vi "ev3-samplecollector.vi"() -> ()   [LabVIEW 2013]
uses:
  <vilib>/Utility/inputDevices.llb/joystickAcquire.vi
  <vilib>/NXT/Dual Mode Library/Sensors/Read_Battery.vi
  <vilib>/NXT/Block Support/NXT_OutputPort.ctl
  <vilib>/NXT/LegoClasses/BrickReference/BrickReference.lvclass
  <vilib>/NXT/Subs/LVHSConnector.ctl
  <vilib>/NXT/NXTIO Xnodes/NXTIONodeSubVIs/NXTMoveMotors.vi
  <vilib>/NXT/NXTIO Xnodes/NXTIOXNode/NXTIO.xnode
  <vilib>/NXT/Dual Mode Library/Sound/Tone.vi
  <vilib>/Utility/inputDevices.llb/closeJoystick.vi
  <vilib>/NXT/NXTIO Xnodes/NXTIONodeSubVIs/NXTStopMotors.vi
  <vilib>/NXT/NXTIO Xnodes/AddressXNode/NXTIOAddress.xnode
  <vilib>/NXT/NXT Controls/ConnectionType.ctl
panel:
  in  "Connection Type":T1=enum."USB"
  in  "NXT/EV3 name":string
  out "throttle":dbl(knob) scale=0.0..100.0
  in  "Stop Button":bool
  out "Battery voltage [V]":sgl(slide) scale=0.0..10.0
  in  "Enable throttle":bool
  out "Voltage":dbl
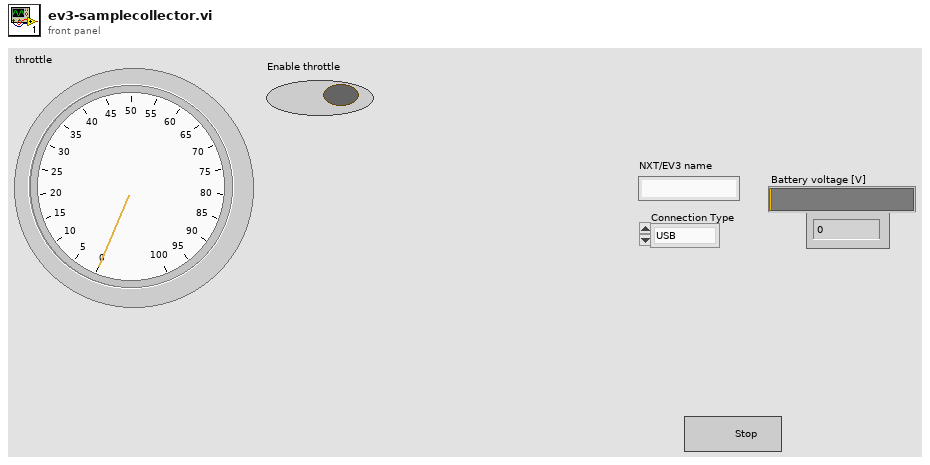
[diagram p1: front panel]
types:
  T1 = typedef "ConnectionType.ctl" = enum16{"Bluetooth", "USB", "WiFi"}
  T2 = typedef "LVHSConnector.ctl" = refnum<class "BrickReference.lvclass">
  T3 = typedef "NXT_OutputPort.ctl" = u8
  T4 = cluster{"X axis":i32, "Y axis":i32, "Z axis":i32, "X axis rotation":i32, "Y axis rotation":i32, "Z axis rotation":i32, "U axis":i32, "V axis":i32}
  T5 = cluster{"button 1":bool, "button 2":bool, "button 3":bool, "button 4":bool, "button 5":bool, "button 6":bool, "button 7":bool, "button 8":bool, "button 9":bool, "button 10":bool, "button 11":bool, "button 12":bool, "button 13":bool, "button 14":bool, "button 15":bool, "button 16":bool, "button 17":bool, "button 18":bool, "button 19":bool, "button 20":bool, "button 21":bool, "button 22":bool, "button 23":bool, "button 24":bool, "button 25":bool, "button 26":bool, "button 27":bool, "button 28":bool, "button 29":bool, "button 30":bool, "button 31":bool, "button 32":bool}
  T6 = cluster{"X axis":dbl, "Y axis":dbl, "Z axis":dbl, "X axis rotation":dbl, "Y axis rotation":dbl, "Z axis rotation":dbl, "U axis":dbl, "V axis":dbl}
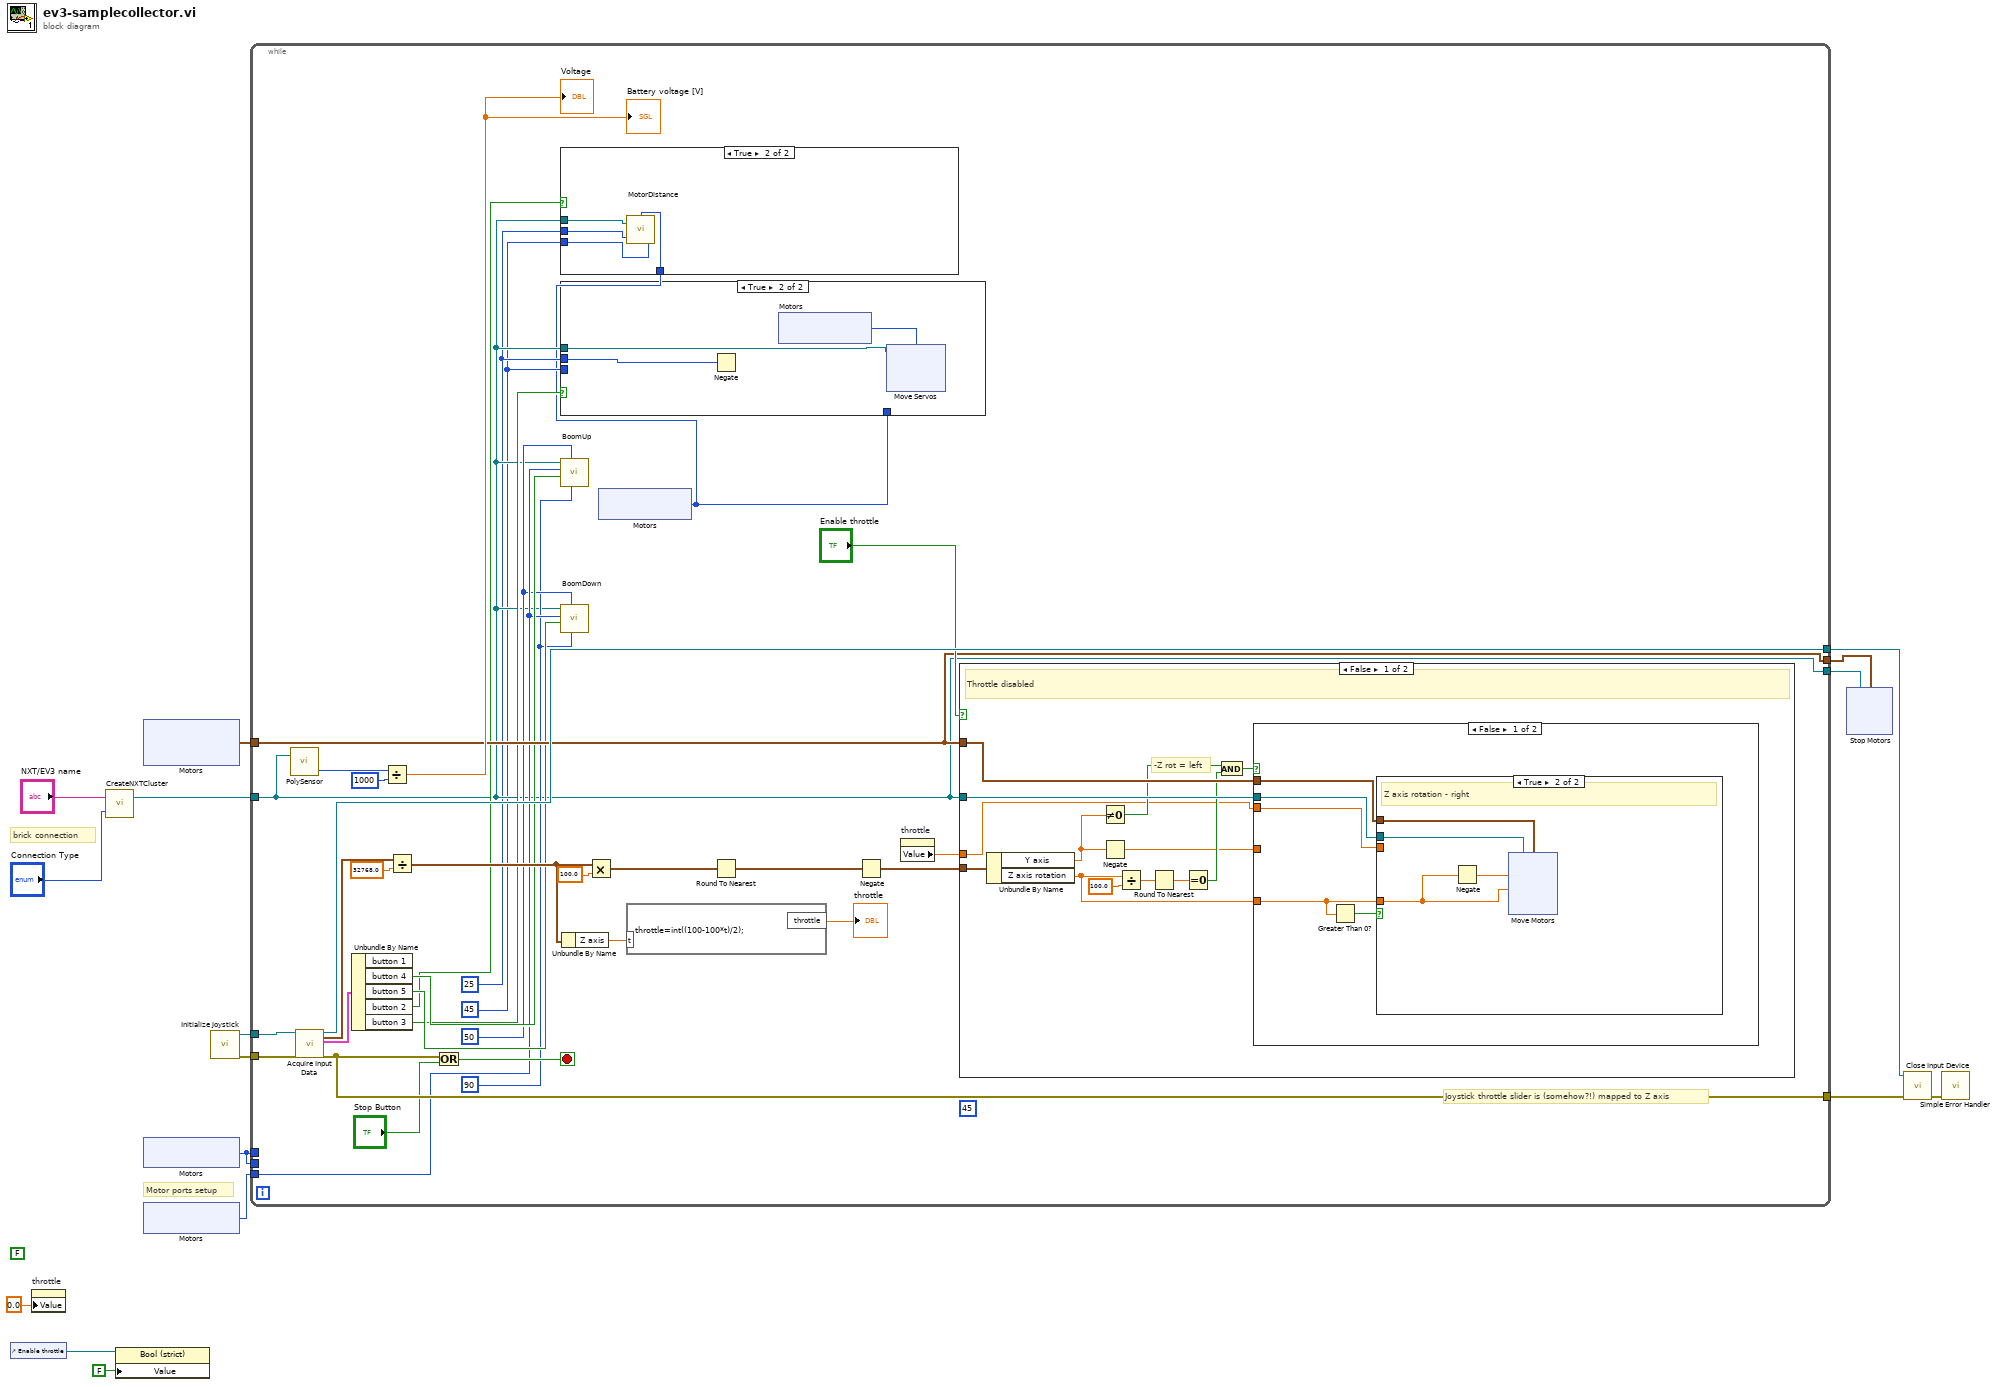
[diagram p0: block diagram]
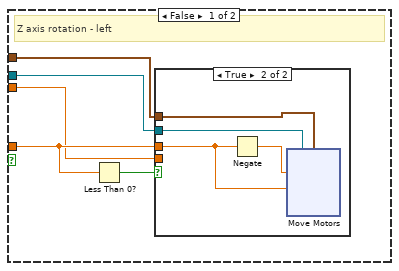
[diagram p4: hidden frame]
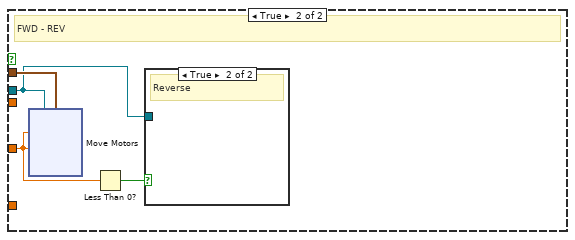
[diagram p6: hidden frame]
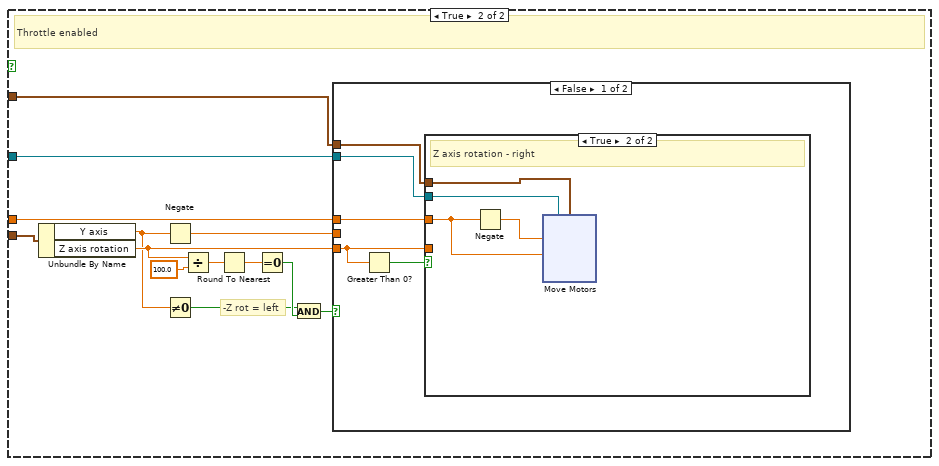
[diagram p8: hidden frame]
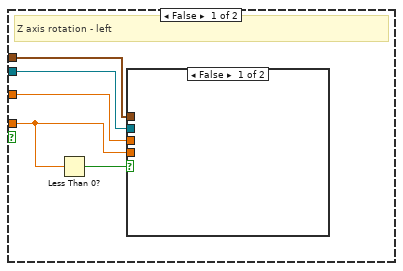
[diagram p9: hidden frame]
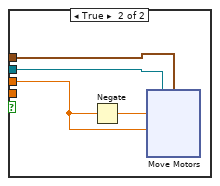
[diagram p10: hidden frame]
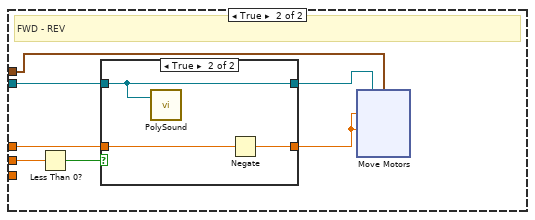
[diagram p11: hidden frame]
diagram:
  (unwired) FALSE ("ClawClosed")
  # "Motor ports setup"
  # "brick connection"
  n1 = control-ref of="Enable throttle"() -> (w7:refnum<vi>)
  n2 = property on="throttle" class="Knob (strict)"("Value"=0.0 ("throttle")) -> ()  [unwired: 2 in, 2 out]
  n3 = call <vilib>:"CreateNXTCluster.vi"("Connection Type"="Connection Type", "NXT/EV3 name"="NXT/EV3 name") -> ("NXT/EV3"=w4:T2)  [unwired: 2 in]
  n4 = property class="Bool (strict)"(reference=w7, "Value"=FALSE) -> ()  [unwired: 1 in, 2 out]
  n5 = xnode "Motors"() -> ("Motor"=w8:cluster{"Port":T3, "Port":T3})
  n6 = xnode "Motors"() -> ("Motor"=w1:T3)
  n7 = xnode "Motors"() -> ("Motor"=w2:T3)
  n8 = call <vilib>:"Initialize Joystick.vi"() -> ("error out"=w15:errorcluster, "device ID"=w16:refnum<k1>)  [unwired: 10 in]
  n9 = while {
    tunnel: w16 -> [w49]
    tunnel: w15 -> [w48]
    tunnel: [w45] -> w14
    tunnel: [w47] -> w13
    tunnel: w4 -> [w20]
    tunnel: [w20] -> w10
    tunnel: [w32] -> w9
    tunnel: w8 -> [w32]
    tunnel: w1 -> [_]
    tunnel: w2 -> [w27]
    tunnel: w1 -> [_]
    stop <- w46 stop-if-true
    w18 = 45 ("Angle of Rotation (360)")
    (unwired) 45 ("Angle of Rotation (360)")
    w19 = 25 ("Claw power")
    w26 = 50 ("Boom motor power")
    w25 = 90 ("Boom Angle of Rotation (360)")
    # "Joystick throttle slider is (somehow?!) mapped to Z axis"
    n10 = call-poly <vilib>:"PolySensor.vi"("NXT/EV3"=w20) -> ("millivolts"=w35:i32)  [unwired: 2 in, 1 out]
    n11 = call-poly <vilib>:"Acquire Input Data.vi"("device ID"=w49, "error in (no error)"=w48) -> ("device ID"=w47:refnum<k1>, "axis info"=w43:T4, "button info"=w30:T5, "error out"=w45:errorcluster)  [unwired: 13 in, 1 out]
    n12 = Unbundle By Name(w30) -> ("button 4"=w29:bool, "button 5"=w28:bool, "button 2"=w22:bool, "button 3"=w21:bool)  [unwired: 1 out]
    n13 = Divide(x=w35, y=1000) -> (x/y=→"Battery voltage [V]" →"Voltage":dbl)
    n14 = Divide(x=w43, y=32768.0) -> (x/y=w39:T6)
    n15 = Or(x=w45, y="Stop Button") -> (x .or. y?=w46:bool)
    n16 = call "BoomUp.vi"("Boom Angle of Rotation (360)"=w25, "Boom motor power"=w26, "button 4"=w29, "Motor"=w27, "BrickReference in"=w20) -> ()  [unwired: 7 in]
    n17 = call "BoomDown.vi"("Boom Angle of Rotation (360)"=w25, "Boom motor power"=w26, "button 5"=w28, "Motor"=w27, "BrickReference in"=w20) -> ()  [unwired: 7 in]
    n18 = Unbundle By Name(w39) -> ("Z axis"=w41:dbl)
    n19 = Multiply(x=w39, y=100.0) -> (x*y=w38:T6)
    n20 = xnode "Motors"() -> ("Motor"=w17:T3)
    n21 = case shown="True" w22 {
      tunnel: w20 -> [_ w58]
      tunnel: w19 -> [_ w57]
      tunnel: w18 -> [_ w56]
      tunnel: w17 -> [_ w55]
      frame False {
      }
      frame True {
        n22 = call <vilib>:"MotorDistance.vi"("Power (75)"=w57, "Angle of Rotation (360)"=w56, "NXT/EV3"=w58, "Output Port (All Ports)"=w55) -> ()  [unwired: 1 out]
      }
    }
    n23 = case shown="True" w21 {
      tunnel: w20 -> [_ w52]
      tunnel: w19 -> [_ w53]
      tunnel: w18 -> [_ _]
      tunnel: w17 -> [_ _]
      frame False {
      }
      frame True {
        n24 = Negate(x=w53) -> ()  [unwired: 1 out]
        n25 = xnode "Motors"() -> ("Motor"=w51:T3)
        n26 = xnode "Move Servos"("Motors"=w51, "NXT/EV3"=w52) -> ()  [unwired: 1 in, 1 out]
      }
    }
    n27 = formula code="throttle=int((100-100*t)/2);"("t"=w41) -> ("throttle"=→"throttle":dbl)
    n28 = Round To Nearest(number=w38) -> (nearest integer value=w24:T6)
    n29 = Negate(x=w24) -> (-x=w23:T6)
    n30 = property on="throttle" class="Knob (strict)"() -> ("Value"=w31:dbl)  [unwired: 2 in, 2 out]
    n31 = case shown="False" "Enable throttle" {
      tunnel: w20 -> [w70 w121]
      tunnel: w23 -> [w71 w120]
      tunnel: w32 -> [w69 w119]
      tunnel: w31 -> [w59 w118]
      frame False {
        # "-Z rot = left"
        # "Throttle disabled"
        n32 = Unbundle By Name(w71) -> ("Y axis"=w61:dbl, "Z axis rotation"=w65:dbl)
        n33 = Not Equal To 0?(x=w61) -> (x != 0?=w66:bool)
        n34 = Negate(x=w61) -> (-x=w60:dbl)
        n35 = Divide(x=w65, y=100.0) -> (x/y=w63:dbl)
        n36 = Round To Nearest(number=w63) -> (nearest integer value=w62:dbl)
        n37 = Equal To 0?(x=w62) -> (x = 0?=w68:bool)
        n38 = And(x=w66, y=w68) -> (x .and. y?=w67:bool)
        n39 = case shown="False" w67 {
          tunnel: w70 -> [w74 w106]
          tunnel: w69 -> [w75 w109]
          tunnel: w60 -> [_ w108]
          tunnel: w65 -> [w73 _]
          tunnel: w59 -> [w72 _]
          frame False {
            n40 = Greater Than 0?(x=w73) -> (x > 0?=w76:bool)
            n41 = case shown="True" w76 {
              tunnel: w75 -> [w79 w97]
              tunnel: w74 -> [w80 w96]
              tunnel: w73 -> [w78 w94]
              tunnel: w72 -> [w77 _]
              frame False {
                # "Z axis rotation - left"
                n42 = Less Than 0?(x=w78) -> (x < 0?=w81:bool)
                n43 = case shown="True" w81 {
                  tunnel: w80 -> [_ w85]
                  tunnel: w79 -> [_ w84]
                  tunnel: w78 -> [_ w82]
                  tunnel: w77 -> [_ _]
                  frame False {
                  }
                  frame True {
                    n44 = Negate(x=w82) -> (-x=w83:dbl)
                    n45 = xnode "Move Motors"("Power/Speed 2"=w82, "Power/Speed 1"=w83, "Motors"=w84, "NXT/EV3"=w85) -> ()  [unwired: 1 out]
                  }
                }
              }
              frame True {
                # "Z axis rotation - right"
                n46 = Negate(x=w94) -> (-x=w95:dbl)
                n47 = xnode "Move Motors"("Power/Speed 2"=w94, "Power/Speed 1"=w95, "Motors"=w97, "NXT/EV3"=w96) -> ()  [unwired: 1 out]
              }
            }
          }
          frame True {
            # "FWD - REV"
            n48 = xnode "Move Motors"("Power/Speed 2"=w108, "Power/Speed 1"=w108, "Motors"=w109, "NXT/EV3"=w106) -> ()  [unwired: 1 out]
            n49 = Less Than 0?(x=w108) -> (x < 0?=w107:bool)
            n50 = case shown="True" w107 {
              tunnel: w106 -> [_ _]
              frame False {
              }
              frame True {
                # "Reverse"
              }
            }
          }
        }
      }
      frame True {
        # "-Z rot = left"
        # "Throttle enabled"
        n51 = Unbundle By Name(w120) -> ("Y axis"=w123:dbl, "Z axis rotation"=w127:dbl)
        n52 = Negate(x=w123) -> (-x=w122:dbl)
        n53 = Not Equal To 0?(x=w123) -> (x != 0?=w128:bool)
        n54 = Divide(x=w127, y=100.0) -> (x/y=w125:dbl)
        n55 = Round To Nearest(number=w125) -> (nearest integer value=w124:dbl)
        n56 = Equal To 0?(x=w124) -> (x = 0?=w130:bool)
        n57 = And(x=w128, y=w130) -> (x .and. y?=w129:bool)
        n58 = case shown="False" w129 {
          tunnel: w121 -> [w133 w169]
          tunnel: w119 -> [w134 w166]
          tunnel: w122 -> [_ w171]
          tunnel: w127 -> [w132 _]
          tunnel: w118 -> [w131 w167]
          frame False {
            n59 = Greater Than 0?(x=w132) -> (x > 0?=w135:bool)
            n60 = case shown="True" w135 {
              tunnel: w134 -> [w138 w156]
              tunnel: w133 -> [w139 w155]
              tunnel: w132 -> [w137 _]
              tunnel: w131 -> [w136 w153]
              frame False {
                # "Z axis rotation - left"
                n61 = Less Than 0?(x=w137) -> (x < 0?=w140:bool)
                n62 = case shown="False" w140 {
                  tunnel: w139 -> [_ w144]
                  tunnel: w138 -> [_ w143]
                  tunnel: w137 -> [_ _]
                  tunnel: w136 -> [_ w141]
                  frame False {
                  }
                  frame True {
                    n63 = Negate(x=w141) -> (-x=w142:dbl)
                    n64 = xnode "Move Motors"("Power/Speed 2"=w141, "Power/Speed 1"=w142, "Motors"=w143, "NXT/EV3"=w144) -> ()  [unwired: 1 out]
                  }
                }
              }
              frame True {
                # "Z axis rotation - right"
                n65 = Negate(x=w153) -> (-x=w154:dbl)
                n66 = xnode "Move Motors"("Power/Speed 2"=w153, "Power/Speed 1"=w154, "Motors"=w156, "NXT/EV3"=w155) -> ()  [unwired: 1 out]
              }
            }
          }
          frame True {
            # "FWD - REV"
            n67 = Less Than 0?(x=w171) -> (x < 0?=w170:bool)
            n68 = case shown="True" w170 {
              tunnel: w169 -> [w172 w176]
              tunnel: [w172 w176] -> w168
              tunnel: w167 -> [w173 w175]
              tunnel: [w173 w174] -> w165
              frame False {
              }
              frame True {
                n69 = call-poly <vilib>:"PolySound.vi"("NXT/EV3"=w176) -> ()  [unwired: 3 in, 1 out]
                n70 = Negate(x=w175) -> (-x=w174:dbl)
              }
            }
            n71 = xnode "Move Motors"("Power/Speed 2"=w165, "Power/Speed 1"=w165, "Motors"=w166, "NXT/EV3"=w168) -> ()  [unwired: 1 out]
          }
        }
      }
    }
  }
  n72 = xnode "Stop Motors"("Motors"=w9, "NXT/EV3"=w10) -> ()  [unwired: 1 out]
  n73 = call-poly <vilib>:"Close Input Device.vi"("error in (no error)"=w14, "device ID"=w13) -> ("error out"=w3:errorcluster)  [unwired: 8 in]
  n74 = call <vilib>:"Simple Error Handler.vi"("error in (no error)"=w3) -> ()  [unwired: 4 in, 5 out]
